vi "Welcome Animation.vi"(8 "error in (no error)":errorcluster, 11 "Controller in":refnum<class "Controller.lvclass">) -> (0 "error out":errorcluster, 3 "Controller out":refnum<class "Controller.lvclass">)   [LabVIEW 2024, in "Controller.lvlib" / "Controller.lvclass"]
uses:
  Controller.lvclass
  Controller.lvclass/Controller.ctl
  MC Screen/Grid Screen Messages/Reset Board Appearance Msg/Reset Board Appearance Msg.lvclass/Reset Board Appearance Msg.ctl
  <vilib>/ActorFramework/Message Enqueuer/Message Enqueuer.lvclass/Message Enqueuer.ctl
  <vilib>/numeric/Random Number (Range) U64.vi
  <vilib>/numeric/sub_Random U32.vi
  <vilib>/ActorFramework/Message Enqueuer/Enqueue.vi
  MC Screen/Grid Screen Messages/Reset Board Appearance Msg/Reset Board Appearance Msg.lvclass
  C:/Program Files/National Instruments/LabVIEW 2024/vi.lib/ActorFramework/Message/Message.lvclass
  Contestant/Contestant Messages/Light to Nuetral Msg/Light to Nuetral Msg.lvclass
  Contestant/Contestant Messages/Light to Red Msg/Light to Red Msg.lvclass
  Contestant/Contestant Messages/Light to Green Msg/Light to Green Msg.lvclass
  <vilib>/ActorFramework/Message Priority Queue/Priority Enqueue.vi
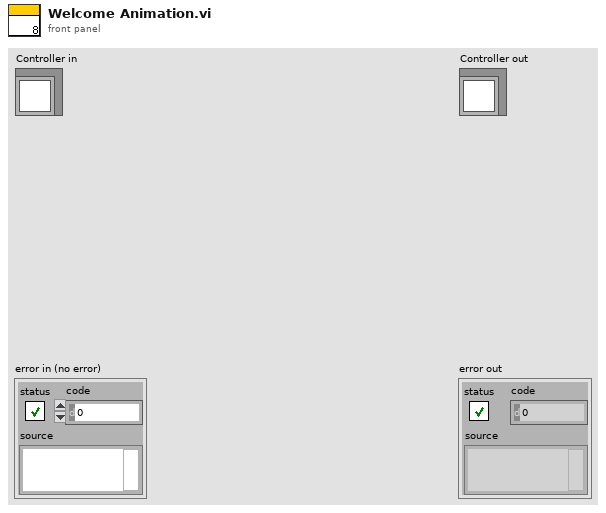
[diagram p1: front panel]
types:
  T1 = map{i32, refnum<class "Message Enqueuer.lvclass">}
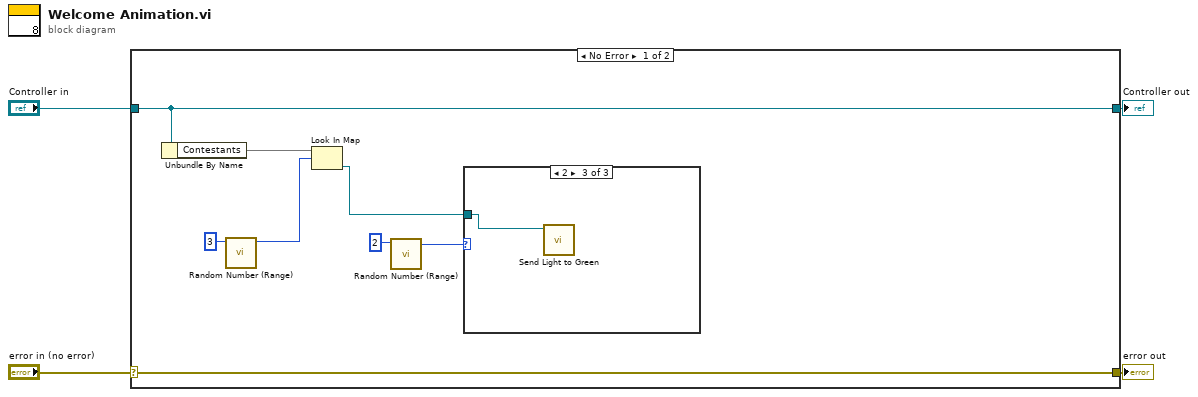
[diagram p0: block diagram]
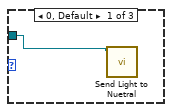
[diagram p2: hidden frame]
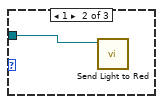
[diagram p3: hidden frame]
diagram:
  n1 = case shown="No Error" "error in (no error)" {
    selector: "error in (no error)" -> [w12 w17]
    tunnel: [w12 w17] -> w3
    tunnel: [w5 w16] -> w1
    tunnel: "Controller in" -> [w5 w16]
    frame No Error {
      n2 = Unbundle By Name(w5) -> ("Contestants"=w11:T1)
      n3 = call-poly <vilib>:"Random Number (Range).vi"("upper bound (100)"=u64 3) -> ("number"=w9:u64)  [unwired: 10 in]
      n4 = Look In Map(map=w11, key=w9) -> (value=w6:refnum<class "Message Enqueuer.lvclass">)  [unwired: 1 in, 1 out]
      n5 = call-poly <vilib>:"Random Number (Range).vi"("upper bound (100)"=u64 2) -> ("number"=w7:u64)  [unwired: 10 in]
      n6 = case shown="2" w7 {
        tunnel: w6 -> [w13 w14 w15]
        frame 0, Default {
          n7 = call "Send Light to Nuetral.vi"("Message Enqueuer"=w13) -> ()  [unwired: 9 in, 2 out]
        }
        frame 1 {
          n8 = call "Send Light to Red.vi"("Message Enqueuer"=w14) -> ()  [unwired: 9 in, 2 out]
        }
        frame 2 {
          n9 = call "Send Light to Green.vi"("Message Enqueuer"=w15) -> ()  [unwired: 9 in, 2 out]
        }
      }
    }
    frame Error {
    }
  }
  "error out" <- w3
  "Controller out" <- w1
